vi "JTAG Init.vi"(8 "error in (no error)":errorcluster, 11 "Power Target Device":bool) -> (0 "error out":errorcluster, 3 "Device Vcc":i32)   [LabVIEW 2010]
panel:
  in  "PC start address":u16=12544 format="%04x"
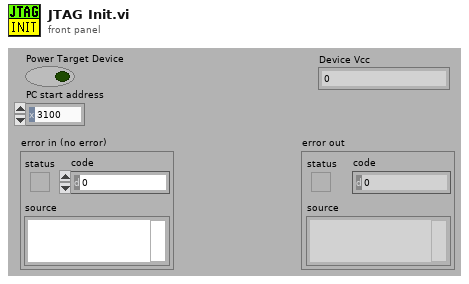
[diagram p1: front panel]
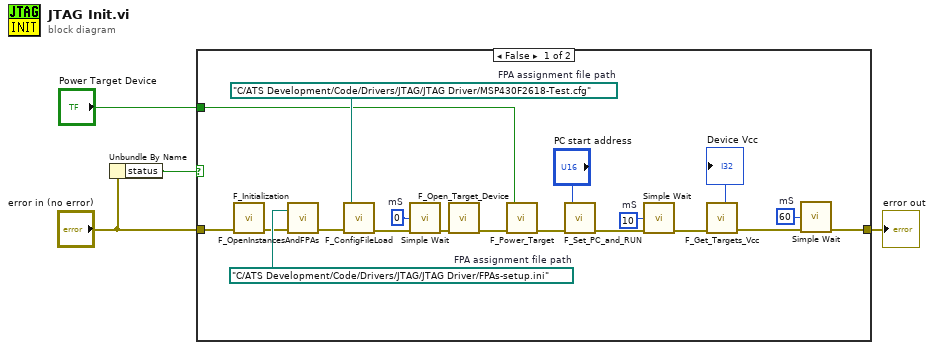
[diagram p0: block diagram]
diagram:
  n1 = Unbundle By Name("error in (no error)") -> ("status"=w4:bool)
  n2 = case shown="False" w4 {
    tunnel: [w5 w24] -> w2
    tunnel: "error in (no error)" -> [w19 w24]
    tunnel: "Power Target Device" -> [w14 _]
    frame False {
      w7 = u32 60  # mS
      w15 = u32 0  # mS
      w18 = u32 10  # mS
      w22 = path "C:/ATS Development/Code/Drivers/JTAG/JTAG Driver/MSP430F2618-Test.cfg"  # FPA assignment file path
      w23 = path "C:/ATS Development/Code/Drivers/JTAG/JTAG Driver/FPAs-setup.ini"  # FPA assignment file path
      n3 = call "F_Initialization.vi"("error in (no error)"=w19) -> ("error out"=w20:errorcluster)
      n4 = call "F_OpenInstancesAndFPAs.vi"("error in (no error)"=w20, "FPA assignment file path"=w23) -> ("error out"=w16:errorcluster)  [unwired: 1 out]
      n5 = call "F_ConfigFileLoad.vi"("error in (no error)"=w16, "Config file path"=w22) -> ("error out"=w12:errorcluster)  [unwired: 1 in]
      n6 = call "Simple Wait.vi"("mS"=w15, "error in"=w12) -> ("error out"=w13:errorcluster)  [unwired: 12 in, 1 out]
      n7 = call "F_Open_Target_Device.vi"("error in (no error)"=w13) -> ("error out"=w9:errorcluster)
      n8 = call "F_Power_Target.vi"("error in (no error)"=w9, "Power Target Device"=w14) -> ("error out"=w8:errorcluster)  [unwired: 1 in]
      n9 = call "F_Set_PC_and_RUN.vi"("error in (no error)"=w8, "PC start address"="PC start address") -> ("error out"=w10:errorcluster)  [unwired: 1 in]
      n10 = call "Simple Wait.vi"("mS"=w18, "error in"=w10) -> ("error out"=w17:errorcluster)  [unwired: 12 in, 1 out]
      n11 = call "F_Get_Targets_Vcc.vi"("error in (no error)"=w17) -> ("error out"=w6:errorcluster, "Device Vcc"=→"Device Vcc":i32)  [unwired: 1 in]
      n12 = call "Simple Wait.vi"("mS"=w7, "error in"=w6) -> ("error out"=w5:errorcluster)  [unwired: 12 in, 1 out]
    }
    frame True {
    }
  }
  "error out" <- w2
